vi "DMC CLI Caraya.vi"() -> ()   [LabVIEW 2023]
uses:
  State Enum.ctl
  <vilib>/Wiresmith Technology/G CLI/CLI Class/CLI.lvclass
  <vilib>/Wiresmith Technology/G CLI/Argument Parser/Option Set Class/Option Set.lvclass
  <vilib>/addons/_JKI Toolkits/Caraya/classes/Test Result/Test Result.lvclass
  <vilib>/Wiresmith Technology/G CLI/Argument Parser/Option Class/Option Configuration.ctl
  <vilib>/Wiresmith Technology/G CLI/Argument Parser/Option Class/Argument Type.ctl
  bceec9fd-d643-4e2c-ae59-84a5c2243fb7.vi
  DMC Folder Test Runner/DMC Folder Test Runner.lvclass
  <vilib>/addons/_JKI Toolkits/Caraya/classes/Test Runner/Read Test VIs.vi
  <vilib>/Wiresmith Technology/G CLI/Argument Parser/Option Class/Option.lvclass
  <vilib>/addons/_JKI Toolkits/Caraya/classes/Test Runner/Test Runner.lvclass
panel:
  out "Test VIs":path[](array[path])
  out "Test Source Paths":path[](array[path])
  out "Verbose":bool
  out "Excluded Bookmarks":string[](array[string])
  out "Included Bookmarks":string[](array[string])
  out "Report Path":path
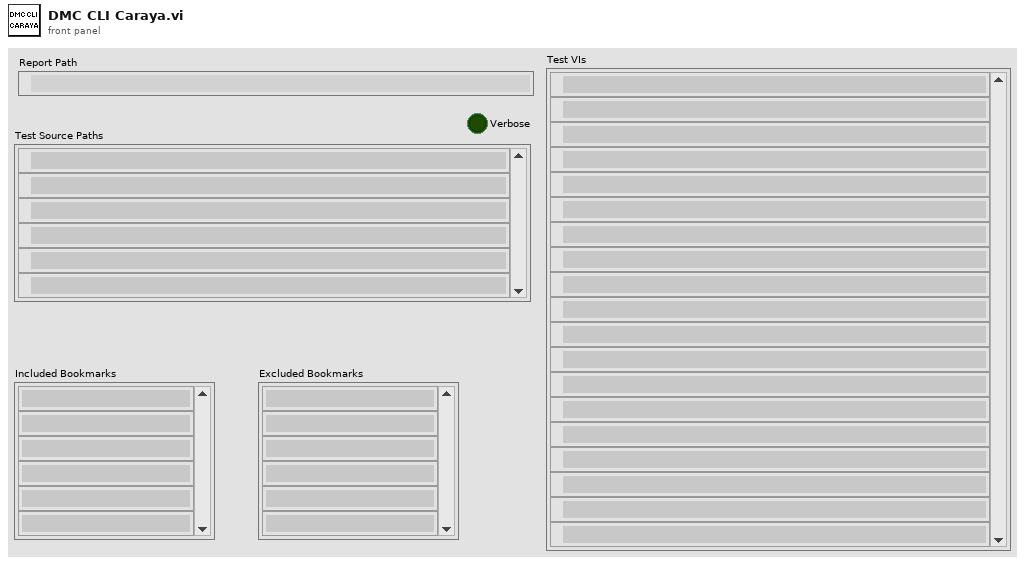
[diagram p1: front panel]
types:
  T1 = cluster{"Report Directory":path, "CLI":refnum<class "CLI.lvclass">, "Option Set":refnum<class "Option Set.lvclass">, "Working Directory":path, "Included Bookmarks":string[], "Excluded Bookmarks":string[], "Verbose":bool, "Report":path, "Source Paths":path[], "Test Suite Results":refnum<class "Test Result.lvclass">, "Pass?":bool, "Test VIs":path[]}
  T2 = typedef "State Enum.ctl" = enum16{"Initialize", "Run Caraya", "Report", "Close", "Help"}
  T3 = typedef "Option Parser.lvlib/Option.lvclass/Option Configuration.ctl" = cluster{"Option Type":T4, "Option Labels":string[], "Key":string, "Description":string, "Required":bool, "Default Value":string}
  T4 = typedef "Option Parser.lvlib/Option.lvclass/Argument Type.ctl" = enum16{"flag", "value"}
  T5 = enum16{"Source", "Report Directory", "Report Name", "Include Bookmarks", "Exclude Bookmarks", "Verbose"}
  T6 = enum16{"Source", "Report Directory", "Report Name", "Include Bookmarks", "Exclude Bookmarks", "Verbose"}[]
  T7 = typedef "Caraya.lvlib/Test Result.lvclass/Node Results (Extended).ctl" = cluster{"Test Node":T8, "Assertions":T10[]}
  T8 = typedef "Caraya.lvlib/Test Result.lvclass/Test Node (Extended).ctl" = cluster{"Test Registration":T9, "Defined":bool, "Passed":bool, "properties":variant}
  T9 = typedef "Caraya.lvlib/Test Result.lvclass/Test Registration Data.ctl" = cluster{"Name":string, "Call Chain":string[], "Time Stamp":timestamp, "Test ID":string, "Caller ID":string}
  T10 = typedef "Caraya.lvlib/Test Result.lvclass/Assert Event Data (Extended).ctl" = cluster{"name":string, "passed":bool, "call-chain":string[], "test-error":errorcluster, "timestamp":timestamp, "assert-id":string, "test-id":string, "time":dbl, "message":string, "properties":variant, "measurements":variant, "user-defined":variant}
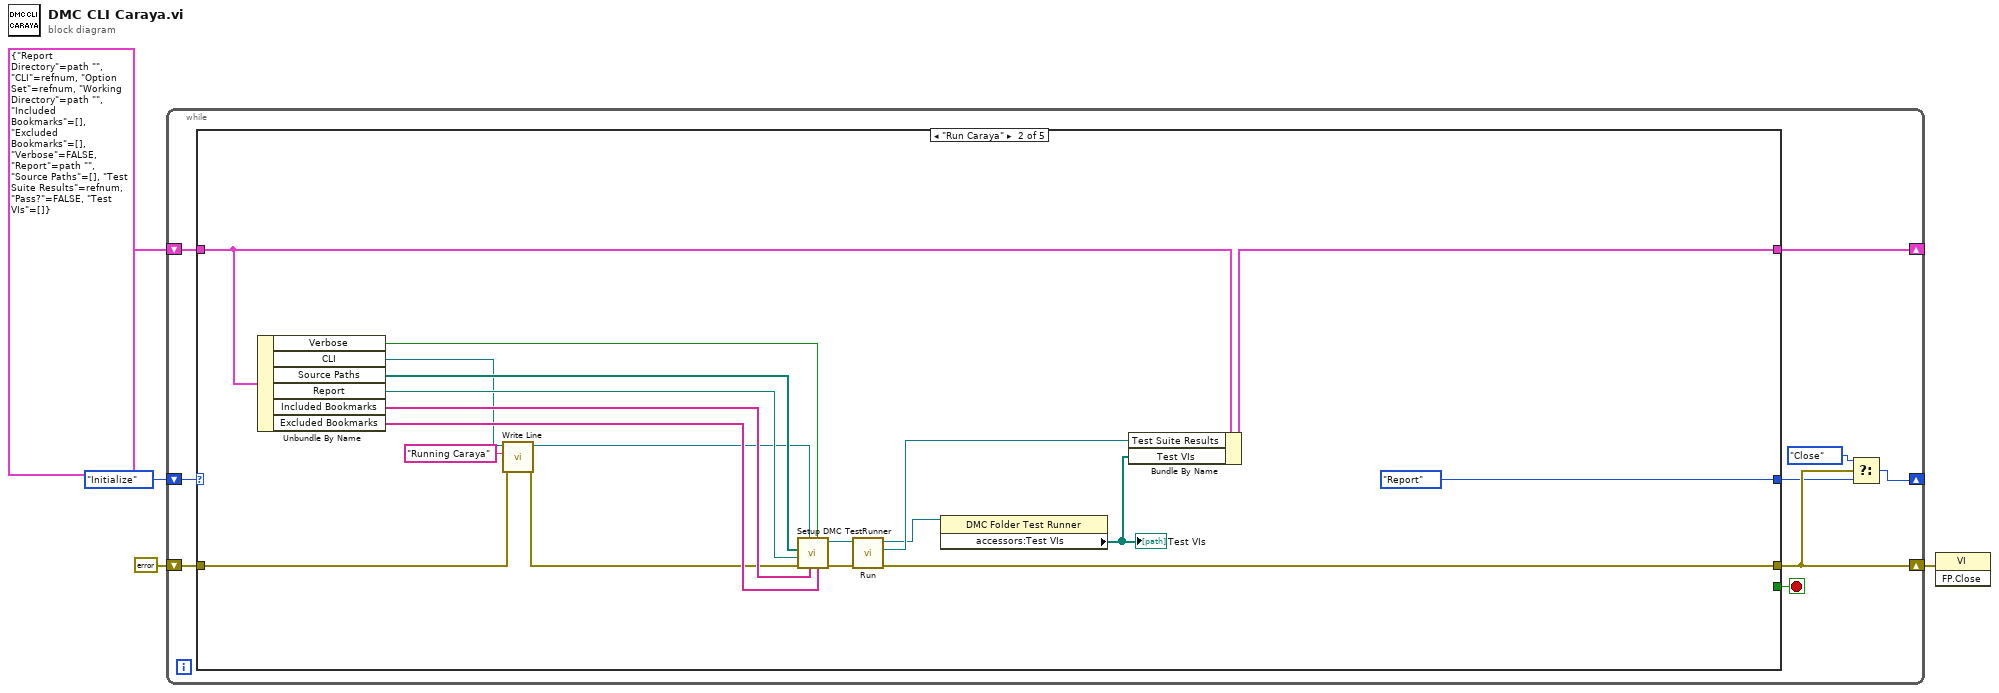
[diagram p0: block diagram]
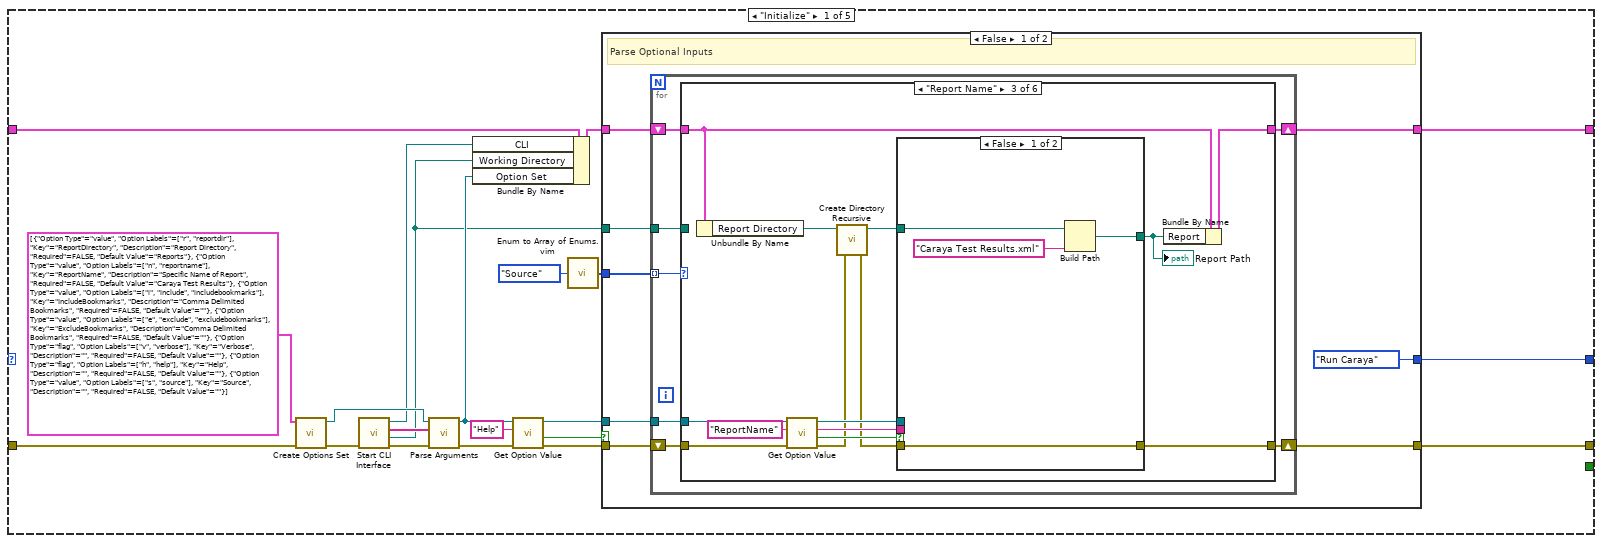
[diagram p2: hidden frame]
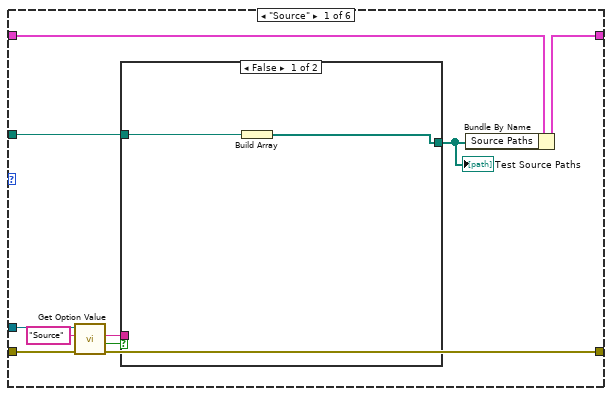
[diagram p3: hidden frame]
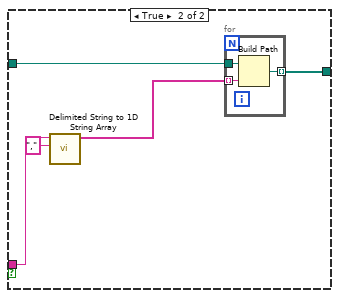
[diagram p4: hidden frame]
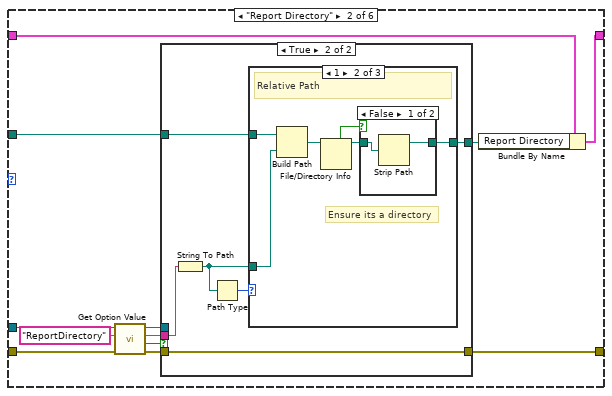
[diagram p5: hidden frame]
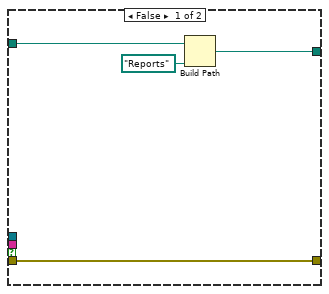
[diagram p6: hidden frame]
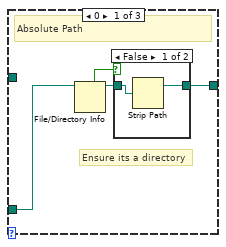
[diagram p7: hidden frame]
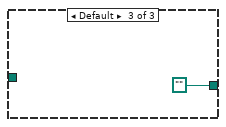
[diagram p10: hidden frame]
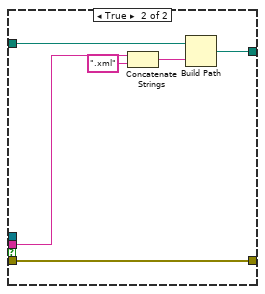
[diagram p11: hidden frame]
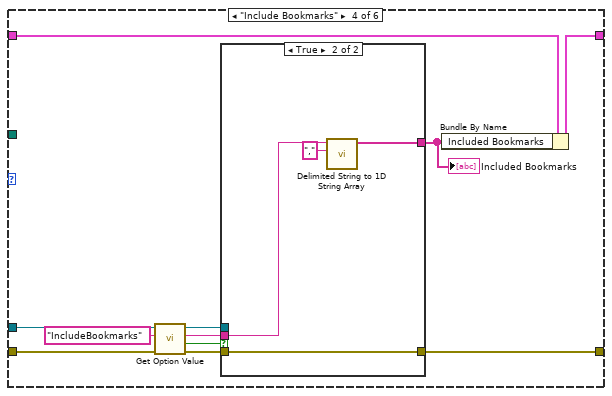
[diagram p12: hidden frame]
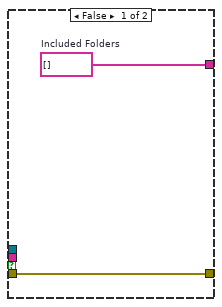
[diagram p13: hidden frame]
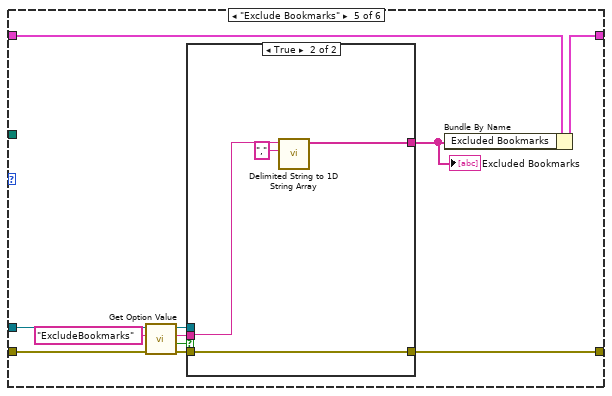
[diagram p14: hidden frame]
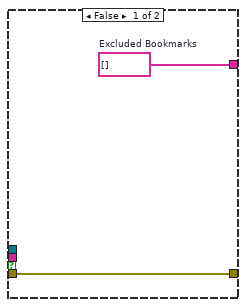
[diagram p15: hidden frame]
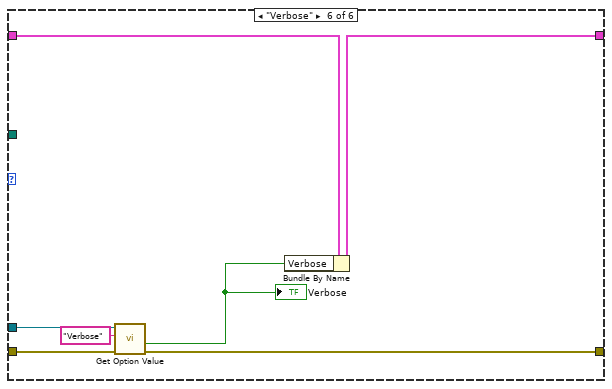
[diagram p16: hidden frame]
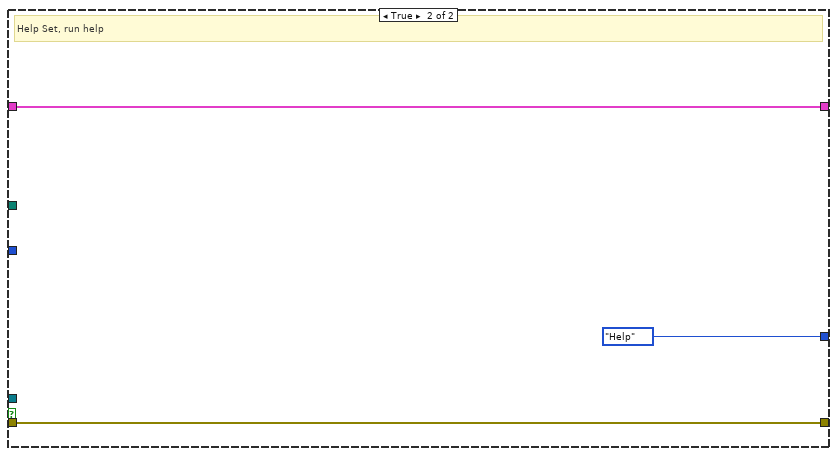
[diagram p17: hidden frame]
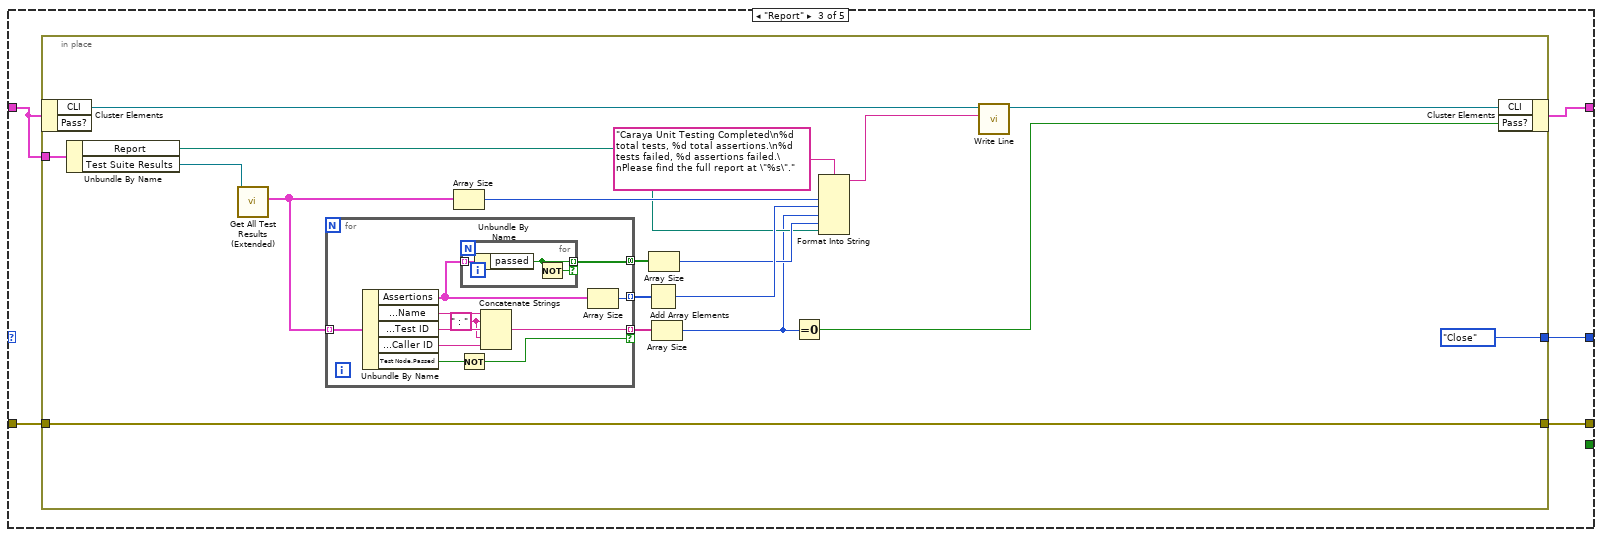
[diagram p18: hidden frame]
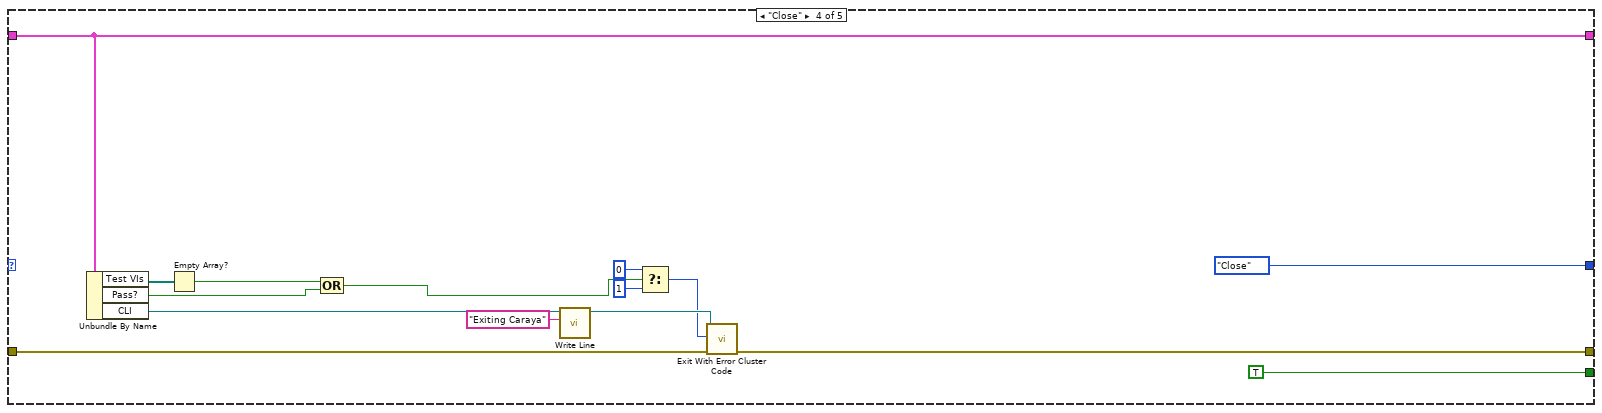
[diagram p19: hidden frame]
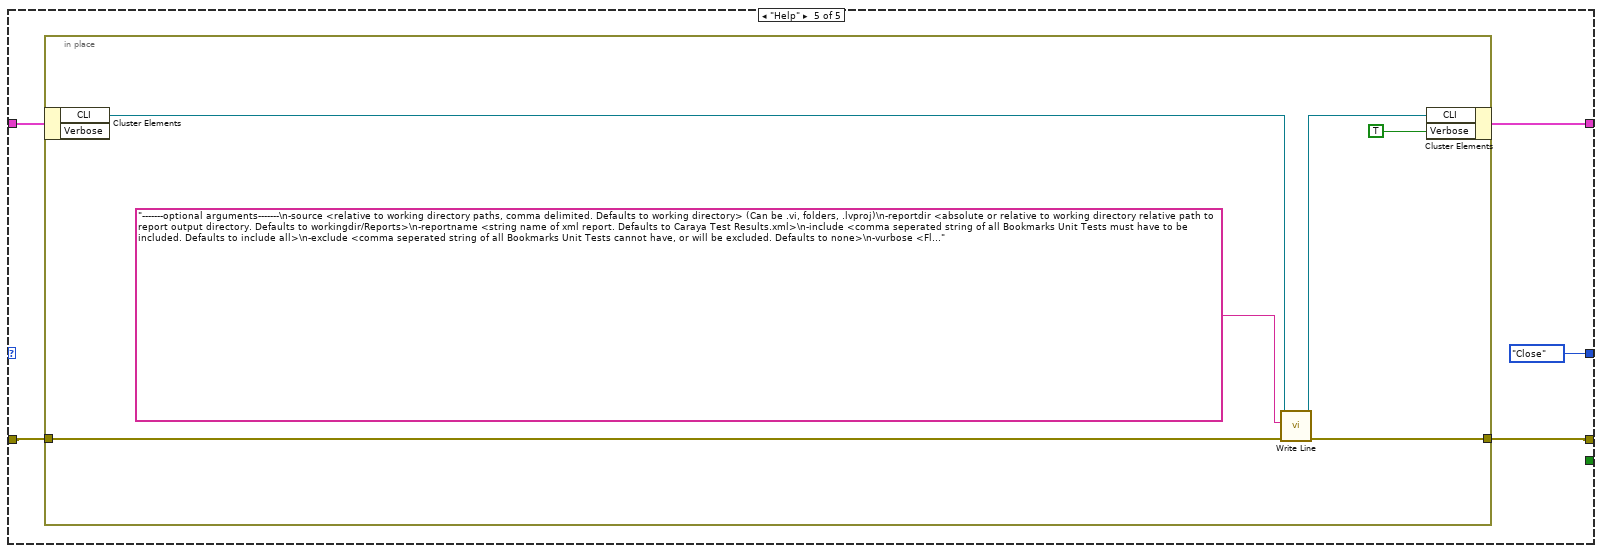
[diagram p20: hidden frame]
diagram:
  n1 = while {
    shift-right: [w6] -> _
    shift-left: State_Enum."Initialize" -> [w13]
    shift-right: [w10] -> _
    shift-left: T1 {"Report Directory"=path "", "CLI"=refnum, "Option Set"=refnum, "Working Directory"=path "", "Included Bookmarks"=[], "Excluded Bookmarks"=[], "Verbose"=FALSE, "Report"=path "", "Source Paths"=[], "Test Suite Results"=refnum, "Pass?"=FALSE, "Test VIs"=[]} -> [w12]
    shift-right: [w9] -> w1
    shift-left: errorcluster {"status"=FALSE, "code"=0, "source"=""} ("error out") -> [w11]
    stop <- w5 stop-if-true
    n2 = case shown="\"Run Caraya\"" w13 {
      tunnel: w12 -> [w34 w194 w196 w247 w249]
      tunnel: w11 -> [w30 w179 w199 w237 w251]
      tunnel: [w15 w186 w200 w247 w248] -> w10
      tunnel: [w19 w184 w198 w246 w250] -> w9
      tunnel: [w33 State_Enum."Report" w197 State_Enum."Close" State_Enum."Close"] -> w7
      tunnel: [_ _ _ TRUE _] -> w5
      frame "Initialize" {
        n3 = call <vilib>:"Create Options Set.vi"("error in (no error)"=w30, "Options"=T3[] [{"Option Type"=enum."value", "Option Labels"=["r", "reportdir"], "Key"="ReportDirectory", "Description"="Report Directory", "Required"=FALSE, "Default Value"="Reports"}, {"Option Type"=enum."value", "Option Labels"=["n", "reportname"], "Key"="ReportName", "Description"="Specific Name of Report", "Required"=FALSE, "Default Value"="Caraya Test Results"}, {"Option Type"=enum."value", "Option Labels"=["i", "include", "includebookmarks"], "Key"="IncludeBookmarks", "Description"="Comma Delimited Bookmarks", "Required"=FALSE, "Default Value"=""}, {"Option Type"=enum."value", "Option Labels"=["e", "exclude", "excludebookmarks"], "Key"="ExcludeBookmarks", "Description"="Comma Delimited Bookmarks", "Required"=FALSE, "Default Value"=""}, {"Option Type"=enum."flag", "Option Labels"=["v", "verbose"], "Key"="Verbose", "Description"="", "Required"=FALSE, "Default Value"=""}, {"Option Type"=enum."flag", "Option Labels"=["h", "help"], "Key"="Help", "Description"="", "Required"=FALSE, "Default Value"=""}, {"Option Type"=enum."value", "Option Labels"=["s", "source"], "Key"="Source", "Description"="", "Required"=FALSE, "Default Value"=""}]) -> ("error out"=w31:errorcluster, "Option Set out"=w29:refnum<class "Option Set.lvclass">)  [unwired: 8 in]
        n4 = call <vilib>:"Start CLI Interface.vi"("error in (no error)"=w31) -> ("error out"=w32:errorcluster, "Working Directory"=w16:path, "Custom Parameters"=w28:string[], "CLI out"=w24:refnum<class "CLI.lvclass">)  [unwired: 7 in]
        n5 = call <vilib>:"Parse Arguments.vi"("error in (no error)"=w32, "Arguments"=w28, "Option Set in"=w29) -> ("error out"=w26:errorcluster, "Option Set out"=w23:refnum<class "Option Set.lvclass">)  [unwired: 5 in, 2 out]
        n6 = Bundle By Name(cluster=w34, "CLI"=w24, "Working Directory"=w16, "Option Set"=w23) -> (w25:T1)
        n7 = call <vilib>:"Get Option Value.vi"("error in (no error)"=w26, "Option Key"="Help", "Option Set in"=w23) -> ("error out"=w21:errorcluster, "Set"=w22:bool, "Option Set out"=w20:refnum<class "Option Set.lvclass">)  [unwired: 5 in, 1 out]
        n8 = call "Enum to Array of Enums.vim"("enum"=T5."Source") -> ("array of enums"=w17:T6)
        n9 = case shown="False" w22 {
          tunnel: [w38 w175] -> w15
          tunnel: [State_Enum."Run Caraya" State_Enum."Help"] -> w33
          tunnel: w25 -> [w40 w175]
          tunnel: w21 -> [w41 w174]
          tunnel: w20 -> [w42 _]
          tunnel: [w36 w174] -> w19
          tunnel: w17 -> [w39 _]
          tunnel: w16 -> [w37 _]
          frame False {
            # "Parse Optional Inputs"
            n10 = for {
              tunnel: w42 -> [w49]
              shift-right: [w46] -> w38
              shift-left: w40 -> [w45]
              tunnel: w39 -> [w47] mode=indexing
              tunnel: w37 -> [w44]
              shift-right: [w43] -> w36
              shift-left: w41 -> [w48]
              n11 = case shown="\"Report Name\"" w47 {
                tunnel: w49 -> [w59 w81 w122 w143 w160 w173]
                tunnel: w48 -> [w58 w80 w121 w142 w159 w172]
                tunnel: [w54 w72 w115 w134 w151 w168] -> w46
                tunnel: w45 -> [w56 w74 w114 w136 w153 w170]
                tunnel: w44 -> [w53 w71 _ _ _ _]
                tunnel: [w55 w73 w116 w135 w152 w169] -> w43
                frame "Source" {
                  n12 = call <vilib>:"Get Option Value.vi"("error in (no error)"=w58, "Option Key"="Source", "Option Set in"=w59) -> ("error out"=w55:errorcluster, "Set"=w50:bool, "Value"=w52:string)  [unwired: 5 in, 1 out]
                  n13 = case shown="False" w50 {
                    tunnel: w53 -> [w61 w64]
                    tunnel: w52 -> [_ w66]
                    tunnel: [w60 w62] -> w51
                    frame False {
                      n14 = Build Array(w61) -> (w60:path[])
                    }
                    frame True {
                      n15 = call <vilib>:"Delimited String to 1D String Array.vi"("delimiter"=",", "delimited string"=w66) -> ("string array"=w63:string[])  [unwired: 9 in]
                      n16 = for {
                        tunnel: w64 -> [w69]
                        tunnel: w63 -> [w68] mode=indexing
                        tunnel: [w67] -> w62 mode=indexing
                        n17 = Build Path(base path=w69, name or relative path=w68) -> (appended path=w67:path)
                      }
                    }
                  }
                  "Test Source Paths" <- w51
                  n18 = Bundle By Name(cluster=w56, "Source Paths"=w51) -> (w54:T1)
                }
                frame "Report Directory" {
                  n19 = call <vilib>:"Get Option Value.vi"("error in (no error)"=w80, "Option Key"="ReportDirectory", "Option Set in"=w81) -> ("error out"=w78:errorcluster, "Set"=w77:bool, "Value"=w75:string, "Option Set out"=w76:refnum<class "Option Set.lvclass">)  [unwired: 5 in]
                  n20 = case shown="True" w77 {
                    tunnel: w78 -> [w84 w90]
                    tunnel: w76 -> [_ _]
                    tunnel: w75 -> [_ w91]
                    tunnel: [w84 w90] -> w73
                    tunnel: [w83 w87] -> w70
                    tunnel: w71 -> [w82 w86]
                    frame False {
                      n21 = Build Path(base path=w82, name or relative path=path "Reports") -> (appended path=w83:path)
                    }
                    frame True {
                      n22 = String To Path(string=w91) -> (path=w88:path)
                      n23 = Path Type(1:w88) -> (0:w89:i16)
                      n24 = case shown="1" w89 {
                        tunnel: w88 -> [w92 w103 _]
                        tunnel: [w93 w100 path ""] -> w87
                        tunnel: w86 -> [_ w104 _]
                        frame 0 {
                          # "Ensure its a directory"
                          # "Absolute Path"
                          n25 = File/Directory Info(path=w92) -> (path out=w95:path, directory=w94:bool)  [unwired: 1 in, 5 out]
                          n26 = case shown="False" w94 {
                            tunnel: w95 -> [w97 w98]
                            tunnel: [w96 w98] -> w93
                            frame False {
                              n27 = Strip Path(path=w97) -> (stripped path=w96:path)  [unwired: 1 out]
                            }
                            frame True {
                            }
                          }
                        }
                        frame 1 {
                          # "Ensure its a directory"
                          # "Relative Path"
                          n28 = Build Path(base path=w104, name or relative path=w103) -> (appended path=w102:path)
                          n29 = File/Directory Info(path=w102) -> (path out=w101:path, directory=w99:bool)  [unwired: 1 in, 5 out]
                          n30 = case shown="False" w99 {
                            tunnel: w101 -> [w106 w107]
                            tunnel: [w105 w107] -> w100
                            frame False {
                              n31 = Strip Path(path=w106) -> (stripped path=w105:path)  [unwired: 1 out]
                            }
                            frame True {
                            }
                          }
                        }
                        frame Default {
                        }
                      }
                    }
                  }
                  n32 = Bundle By Name(cluster=w74, "Report Directory"=w70) -> (w72:T1)
                }
                frame "Report Name" {
                  n33 = Unbundle By Name(w114) -> ("Report Directory"=w112:path)
                  n34 = call <vilib>:"Get Option Value.vi"("error in (no error)"=w121, "Option Key"="ReportName", "Option Set in"=w122) -> ("error out"=w110:errorcluster, "Set"=w119:bool, "Value"=w117:string, "Option Set out"=w118:refnum<class "Option Set.lvclass">)  [unwired: 5 in]
                  n35 = call <vilib>:"Create Directory Recursive.vi"("error in (no error)"=w110, "directory"=w112) -> ("error out"=w109:errorcluster, "directory copy"=w111:path)  [unwired: 3 in, 1 out]
                  n36 = case shown="False" w119 {
                    tunnel: w109 -> [w126 w132]
                    tunnel: w118 -> [_ _]
                    tunnel: w117 -> [_ w128]
                    tunnel: [w126 w132] -> w116
                    tunnel: [w125 w130] -> w113
                    tunnel: w111 -> [w124 w131]
                    frame False {
                      n37 = Build Path(base path=w124, name or relative path="Caraya Test Results.xml") -> (appended path=w125:path)
                    }
                    frame True {
                      n38 = Concatenate Strings(w128, ".xml" ("string")) -> (w127:string)
                      n39 = Build Path(base path=w131, name or relative path=w127) -> (appended path=w130:path)
                    }
                  }
                  "Report Path" <- w113
                  n40 = Bundle By Name(cluster=w114, "Report"=w113) -> (w115:T1)
                }
                frame "Include Bookmarks" {
                  n41 = call <vilib>:"Get Option Value.vi"("error in (no error)"=w142, "Option Key"="IncludeBookmarks", "Option Set in"=w143) -> ("error out"=w140:errorcluster, "Set"=w139:bool, "Value"=w137:string, "Option Set out"=w138:refnum<class "Option Set.lvclass">)  [unwired: 5 in]
                  n42 = case shown="True" w139 {
                    tunnel: w140 -> [w145 w149]
                    tunnel: w138 -> [_ _]
                    tunnel: w137 -> [_ w147]
                    tunnel: [w145 w149] -> w135
                    tunnel: [w144 w148] -> w133
                    frame False {
                      w144 = string[] []  # Included Folders
                    }
                    frame True {
                      n43 = call <vilib>:"Delimited String to 1D String Array.vi"("delimiter"=",", "delimited string"=w147) -> ("string array"=w148:string[])  [unwired: 9 in]
                    }
                  }
                  "Included Bookmarks" <- w133
                  n44 = Bundle By Name(cluster=w136, "Included Bookmarks"=w133) -> (w134:T1)
                }
                frame "Exclude Bookmarks" {
                  n45 = call <vilib>:"Get Option Value.vi"("error in (no error)"=w159, "Option Key"="ExcludeBookmarks", "Option Set in"=w160) -> ("error out"=w157:errorcluster, "Set"=w156:bool, "Value"=w154:string, "Option Set out"=w155:refnum<class "Option Set.lvclass">)  [unwired: 5 in]
                  n46 = case shown="True" w156 {
                    tunnel: w157 -> [w162 w166]
                    tunnel: w155 -> [_ _]
                    tunnel: w154 -> [_ w164]
                    tunnel: [w162 w166] -> w152
                    tunnel: [w161 w165] -> w150
                    frame False {
                      w161 = string[] []  # Excluded Bookmarks
                    }
                    frame True {
                      n47 = call <vilib>:"Delimited String to 1D String Array.vi"("delimiter"=",", "delimited string"=w164) -> ("string array"=w165:string[])  [unwired: 9 in]
                    }
                  }
                  "Excluded Bookmarks" <- w150
                  n48 = Bundle By Name(cluster=w153, "Excluded Bookmarks"=w150) -> (w151:T1)
                }
                frame "Verbose" {
                  n49 = call <vilib>:"Get Option Value.vi"("error in (no error)"=w172, "Option Key"="Verbose", "Option Set in"=w173) -> ("error out"=w169:errorcluster, "Set"=w167:bool)  [unwired: 5 in, 2 out]
                  "Verbose" <- w167
                  n50 = Bundle By Name(cluster=w170, "Verbose"=w167) -> (w168:T1)
                }
              }
            }
          }
          frame True {
            # "Help Set, run help"
          }
        }
      }
      frame "Run Caraya" {
        n51 = Unbundle By Name(w194) -> ("Verbose"=w193:bool, "CLI"=w183:refnum<class "CLI.lvclass">, "Source Paths"=w192:path[], "Report"=w191:path, "Included Bookmarks"=w190:string[], "Excluded Bookmarks"=w189:string[])
        n52 = call <vilib>:"Write Line.vi"("error in (no error)"=w179, "Text to Write"="Running Caraya", "CLI in"=w183) -> ("error out"=w180:errorcluster, "CLI out"=w182:refnum<class "CLI.lvclass">)  [unwired: 7 in]
        n53 = call "Setup DMC TestRunner.vi"("Exclude Bookmarks"=w189, "Verbose"=w193, "Include Bookmarks"=w190, "CLI"=w182, "error in (no error)"=w180, "Report Path"=w191, "Paths"=w192) -> ("error out"=w187:errorcluster, "DMC Test Runner.Folder out"=w188:refnum<class "DMC Folder Test Runner.lvclass">)  [unwired: 3 in]
        n54 = call <vilib>:"Run.vi"("error in (no error)"=w187, "Test Runner in"=w188) -> ("error out"=w184:errorcluster, "Test Suite Results"=w185:refnum<class "Test Result.lvclass">, "Test Runner out"=w178:refnum<class "DMC Folder Test Runner.lvclass">)  [unwired: 7 in]
        n55 = property class="DMC Folder Test Runner"(reference=w178) -> ("accessors:Test VIs"=w177:path[])  [unwired: 1 in, 2 out]
        "Test VIs" <- w177
        n56 = Bundle By Name(cluster=w194, "Test Suite Results"=w185, "Test VIs"=w177) -> (w186:T1)
      }
      frame "Report" {
        n57 = in-place {
          in-place-border: w199 -> [w202]
          in-place-border: [w202] -> w198
          in-place-border: [State_Enum."Close"] -> w197
          in-place-border: w196 -> [w217]
          n58 = in-place-cluster #1(w196) -> ("CLI"=w205:refnum<class "CLI.lvclass">)  [unwired: 1 out]
          n59 = Unbundle By Name(w217) -> ("Report"=w207:path, "Test Suite Results"=w212:refnum<class "Test Result.lvclass">)
          n60 = call <vilib>:"Get All Test Results (Extended).vi"("Test Result in"=w212) -> ("Test Results"=w211:T7[])  [unwired: 8 in, 2 out]
          n61 = for {
            tunnel: w211 -> [w223] mode=indexing
            tunnel: [w222] -> w210 mode=concatenating
            tunnel: [w221] -> w209 mode=indexing
            tunnel: [w220] -> w208 mode=indexing if=w219
            w226 = " : " ("string")
            n62 = Unbundle By Name(w223) -> ("Assertions"=w224:T10[], "Test Node.Test Registration.Name"=w229:string, "Test Node.Test Registration.Test ID"=w228:string, "Test Node.Test Registration.Caller ID"=w227:string, "Test Node.Passed"=w225:bool)
            n63 = Not(x=w225) -> (.not. x?=w219:bool)
            n64 = for {
              tunnel: w224 -> [w232] mode=indexing
              tunnel: [w231] -> w222 mode=indexing if=w230
              n65 = Unbundle By Name(w232) -> ("passed"=w231:bool)
              n66 = Not(x=w231) -> (.not. x?=w230:bool)
            }
            n67 = Concatenate Strings(w229, w226, w228, w226, w227) -> (w220:string)
            n68 = Array Size(array=w224) -> (size(s)=w221:i32)
          }
          n69 = Array Size(array=w211) -> (size(s)=w215:i32)
          n70 = Add Array Elements(numeric array=w209) -> (sum=w214:i32)
          n71 = Array Size(array=w210) -> (size(s)=w213:i32)
          n72 = Array Size(array=w208) -> (size(s)=w206:i32)
          n73 = Equal To 0?(x=w206) -> (x = 0?=w201:bool)
          n74 = Format Into String(format string="Caraya Unit Testing Completed\n%d total tests, %d total assertions.\n%d tests failed, %d assertions failed.\nPlease find the full report at \"%s\".", w215, w214, w206, w213, w207) -> (resulting string=w203:string)  [unwired: 2 in, 1 out]
          n75 = call <vilib>:"Write Line.vi"("Text to Write"=w203, "CLI in"=w205) -> ("CLI out"=w204:refnum<class "CLI.lvclass">)  [unwired: 8 in, 1 out]
          n76 = in-place-cluster #1("CLI"=w204, "Pass?"=w201) -> (w200:T1)
        }
      }
      frame "Close" {
        n77 = Unbundle By Name(w247) -> ("Test VIs"=w236:path[], "Pass?"=w234:bool, "CLI"=w244:refnum<class "CLI.lvclass">)
        n78 = Empty Array?(array=w236) -> (empty?=w235:bool)
        n79 = Compound Arithmetic op=OR(w235, w234) -> (w233:bool)
        n80 = call <vilib>:"Write Line.vi"("Text to Write"="Exiting Caraya", "CLI in"=w244) -> ("CLI out"=w243:refnum<class "CLI.lvclass">)  [unwired: 8 in, 1 out]
        n81 = Select(t=0, s=w233, f=1 ("No Error Code (0)")) -> (s? t:f=w239:i32)
        n82 = call <vilib>:"Exit With Error Cluster Code.vi"("error in (no error)"=w237, "No Error Code (0)"=w239, "CLI in"=w243) -> ("error out"=w246:errorcluster)  [unwired: 8 in]
      }
      frame "Help" {
        n83 = in-place {
          in-place-border: w251 -> [w258]
          in-place-border: [w257] -> w250
          n84 = in-place-cluster #2(w249) -> ("CLI"=w256:refnum<class "CLI.lvclass">)  [unwired: 1 out]
          n85 = call <vilib>:"Write Line.vi"("error in (no error)"=w258, "Text to Write"="-------optional arguments-------\n-source <relative to working directory paths, comma delimited. Defaults to working directory> (Can be .vi, folders, .lvproj)\n-reportdir <absolute or relative to working directory relative path to report output directory. Defaults to workingdir/Reports>\n-reportname <string name of xml report. Defaults to Caraya Test Results.xml>\n-include <comma seperated string of all Bookmarks Unit Tests must have to be included. Defaults to include all>\n-exclude <comma seperated string of all Bookmarks Unit Tests cannot have, or will be excluded. Defaults to none>\n-vurbose <Flag to set report verbose>\n-help <Returns this help information>" ("string"), "CLI in"=w256) -> ("error out"=w257:errorcluster, "CLI out"=w255:refnum<class "CLI.lvclass">)  [unwired: 7 in]
          n86 = in-place-cluster #2("CLI"=w255, "Verbose"=TRUE ("Threshold Pass")) -> (w248:T1)
        }
      }
    }
    n87 = Select(t=State_Enum."Close", s=w9, f=w7) -> (s? t:f=w6:T2)
  }
  n88 = invoke class="VI" method="FP.Close"(error in=w1) -> ()  [unwired: 2 in, 3 out]
